vi "Init.vi"(8 "error in (no error)":errorcluster, 10 "Enqueuer":refnum<class "Message Enqueuer.lvclass">) -> (0 "error out":errorcluster, 3 "MuxAPI out":refnum<class "MuxAPI.lvclass">)   [LabVIEW 2022 SP3, in "VideoMux.lvlib" / "MuxAPI.lvclass"]
uses:
  MuxAPI.lvclass
  MuxAPI.lvclass/MuxAPI.ctl
  <vilib>/ActorFramework/Message Enqueuer/Message Enqueuer.lvclass
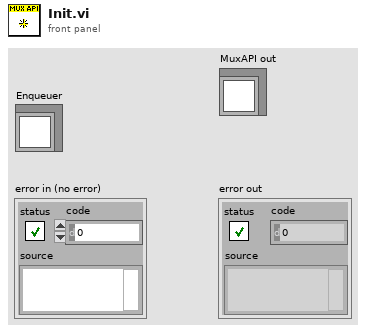
[diagram p1: front panel]
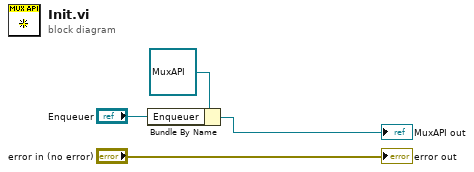
[diagram p0: block diagram]
diagram:
  n1 = Bundle By Name(cluster=refnum<class "MuxAPI.lvclass"> refnum ("MuxAPI in"), "Enqueuer"="Enqueuer") -> (→"MuxAPI out":refnum<class "MuxAPI.lvclass">)
  "error out" <- "error in (no error)"
